vi "Overlay.vi"(8 "error in (no error)":errorcluster, 10 "Image In":T1, 11 "Overlay Base in":refnum<class "Analyze Results Fluence.lvclass">) -> (0 "error out":errorcluster, 2 "Image out":T1, 3 "Overlay Base out":refnum<class "Analyze Results Fluence.lvclass">)   [LabVIEW 2020, in "Analyze Results Fluence.lvclass"]
uses:
  Analyze Results Fluence.lvclass
  C:/POLARIS Programme/POLARIS-AS-3-Cams/Submodules/HIJ Vision/Analyze/Results and Overlays/Results Base/Analyze Results Base.lvclass
  <vilib>/vision/Image Controls.llb/IMAQ Image.ctl
  Results Base/Analyze Results Base.lvclass/Analyze Results Base.ctl
  Results Base/Read Overlay_.vi
  Results Base/Read Overlay colors.vi
  Results Base/Read Font, Size & Style.vi
  Results Base/Analyze Results Base.lvclass
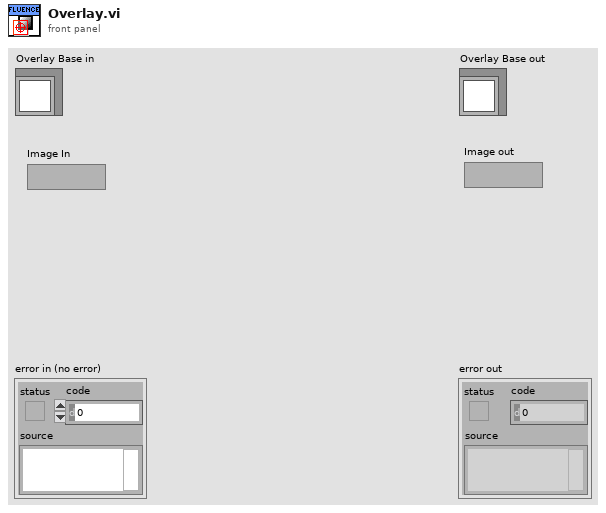
[diagram p1: front panel]
types:
  T1 = typedef "IMAQ Image.ctl" = refnum<image>
  T2 = cluster{"Desired Font (Application)":enum16{"User-specified Font", "Application Font", "System Font", "Dialog Font"}, "[User-specified Font]":cluster{"Font Name":string, "Size":i16, "Strikeout?":bool, "Italic?":bool, "Underline?":bool, "Outline?":bool, "Shadow?":bool, "Bold?":bool, "Rotation Angle":dbl}, "Horizontal Alignment":i16, "Vertical Alignment":i16}
  T3 = typedef "Analyze.lvlib/Analyze Fluence.lvclass/Fluence Info.ctl" = cluster{"Fluence J/cm^2":dbl[unit], "Energy in Area":dbl[unit], "max value":i64, "Max fluence area":cluster{"Left":i32, "Top":i32, "Right":i32, "Bottom":i32}}
  T4 = cluster{"Left":i32, "Top":i32, "Right":i32, "Bottom":i32}
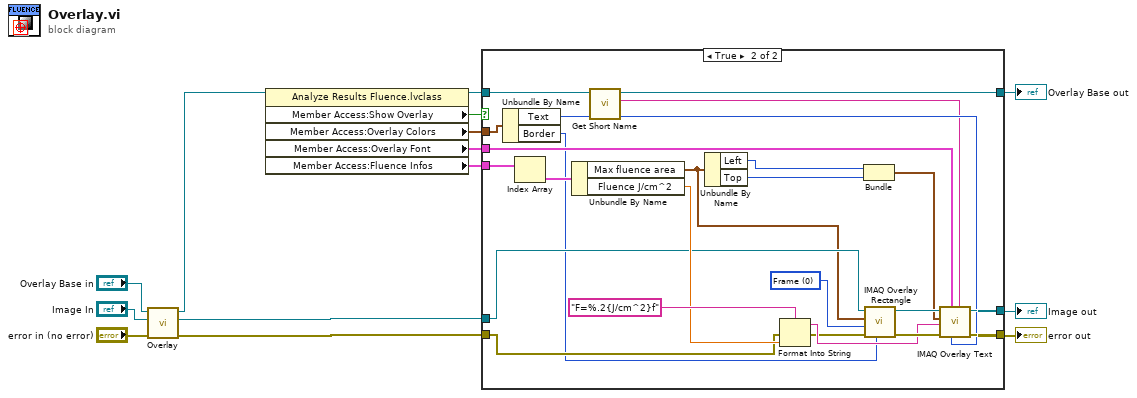
[diagram p0: block diagram]
diagram:
  n1 = call-parent "Overlay.vi"("error in (no error)"="error in (no error)", "Image In"="Image In", "Overlay Base in"="Overlay Base in") -> ("error out"=w5:errorcluster, "Image out"=w7:T1, "Overlay Base out"=w14:refnum<class "Analyze Results Fluence.lvclass">)  [unwired: 6 in]
  n2 = property class="Analyze Results Fluence.lvclass"(reference=w14) -> (reference out=w2:refnum<class "Analyze Results Fluence.lvclass">, "Member Access:Show Overlay"=w10:bool, "Member Access:Overlay Colors"=w8:cluster{"Border":u32, "Text":u32}, "Member Access:Overlay Font"=w3:T2, "Member Access:Fluence Infos"=w9:T3[])  [unwired: 1 in, 1 out]
  n3 = case shown="True" w10 {
    tunnel: [w17 w41] -> w4
    tunnel: w9 -> [_ w35]
    tunnel: w8 -> [_ w33]
    tunnel: w7 -> [w16 w31]
    tunnel: [w16 w30] -> w6
    tunnel: w5 -> [w17 w29]
    tunnel: w3 -> [_ w27]
    tunnel: w2 -> [w15 w20]
    tunnel: [w15 w19] -> w1
    frame False {
    }
    frame True {
      w38 = u32 0 items=["Frame", "Fill", "Highlight"] ("Drawing Mode (Frame)")
      n4 = Unbundle By Name(w33) -> ("Text"=w26:u32, "Border"=w25:u32)
      n5 = Index Array(array=w35) -> (element=w34:T3)  [unwired: 1 in]
      n6 = Unbundle By Name(w34) -> ("Max fluence area"=w24:T4, "Fluence J/cm^2"=w32:dbl[unit])
      n7 = call-dynamic "Get Short Name.vi"("Analyze Results Base in"=w20) -> ("Short Name"=w18:string, "Analyze Results Base out"=w19:refnum<class "Analyze Results Fluence.lvclass">)  [unwired: 8 in, 1 out]
      n8 = Unbundle By Name(w24) -> ("Left"=w23:i32, "Top"=w22:i32)
      n9 = Format Into String(format string="F=%.2{J/cm^2}f", error in=w29, w32) -> (resulting string=w36:string, error out=w28:errorcluster)  [unwired: 1 in]
      n10 = Bundle("Left"=w23, "Top"=w22) -> (w21:cluster{"Left":i32, "Top":i32})  [unwired: 1 in]
      n11 = call "IMAQ Overlay Rectangle"("Color"=w25, "error in (no error)"=w28, "Drawing Mode (Frame)"=w38, "Rectangle"=w24, "Image"=w31) -> ("error out"=w40:errorcluster, "Image Out"=w39:T1)  [unwired: 5 in]
      n12 = call "IMAQ Overlay Text"("Group"=w18, "Text Color (black)"=w26, "Font, Size & Style"=w27, "error in (no error)"=w40, "String"=w36, "Origin"=w21, "Image"=w39) -> ("error out"=w41:errorcluster, "Image Out"=w30:T1)  [unwired: 3 in]
    }
  }
  "error out" <- w4
  "Overlay Base out" <- w1
  "Image out" <- w6
